vi "safeties.vi"() -> ()   [LabVIEW 2014]
uses:
  typedefs/safety data/h-drive teleop safety data.ctl
  typedefs/safety data/container arm safety data.ctl
  typedefs/safety data/lift safety data.ctl
panel:
  in  "Lift PID":T1
  in  "Container Arm PID":T2
  in  "H-Drive PID - Teleop":T3
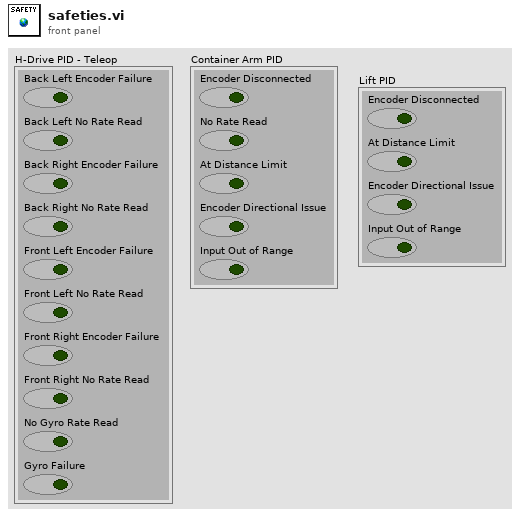
[diagram p1: front panel]
types:
  T1 = typedef "lift safety data.ctl" = cluster{"Encoder Disconnected":bool, "At Distance Limit":bool, "Encoder Directional Issue":bool, "Input Out of Range":bool}
  T2 = typedef "container arm safety data.ctl" = cluster{"Encoder Disconnected":bool, "No Rate Read":bool, "At Distance Limit":bool, "Encoder Directional Issue":bool, "Input Out of Range":bool}
  T3 = typedef "h-drive teleop safety data.ctl" = cluster{"Back Left Encoder Failure":bool, "Back Left No Rate Read":bool, "Back Right Encoder Failure":bool, "Back Right No Rate Read":bool, "Front Left Encoder Failure":bool, "Front Left No Rate Read":bool, "Front Right Encoder Failure":bool, "Front Right No Rate Read":bool, "No Gyro Rate Read":bool, "Gyro Failure":bool}
diagram:
